vi "Read Spreadsheet Settings all.vi"(11 "Select Data Source":enum16{"auto.csv", "Robot Main"}(ring)) -> (3 "Autonomous Data":T1(array[cluster]))   [LabVIEW 2017]
uses:
  Framework/Robot Global Data.vi
  <vilib>/Utility/file.llb/Read Delimited Spreadsheet (string).vi
panel:
  out "error out":errorcluster
  out "all rows":string[][](array[string])
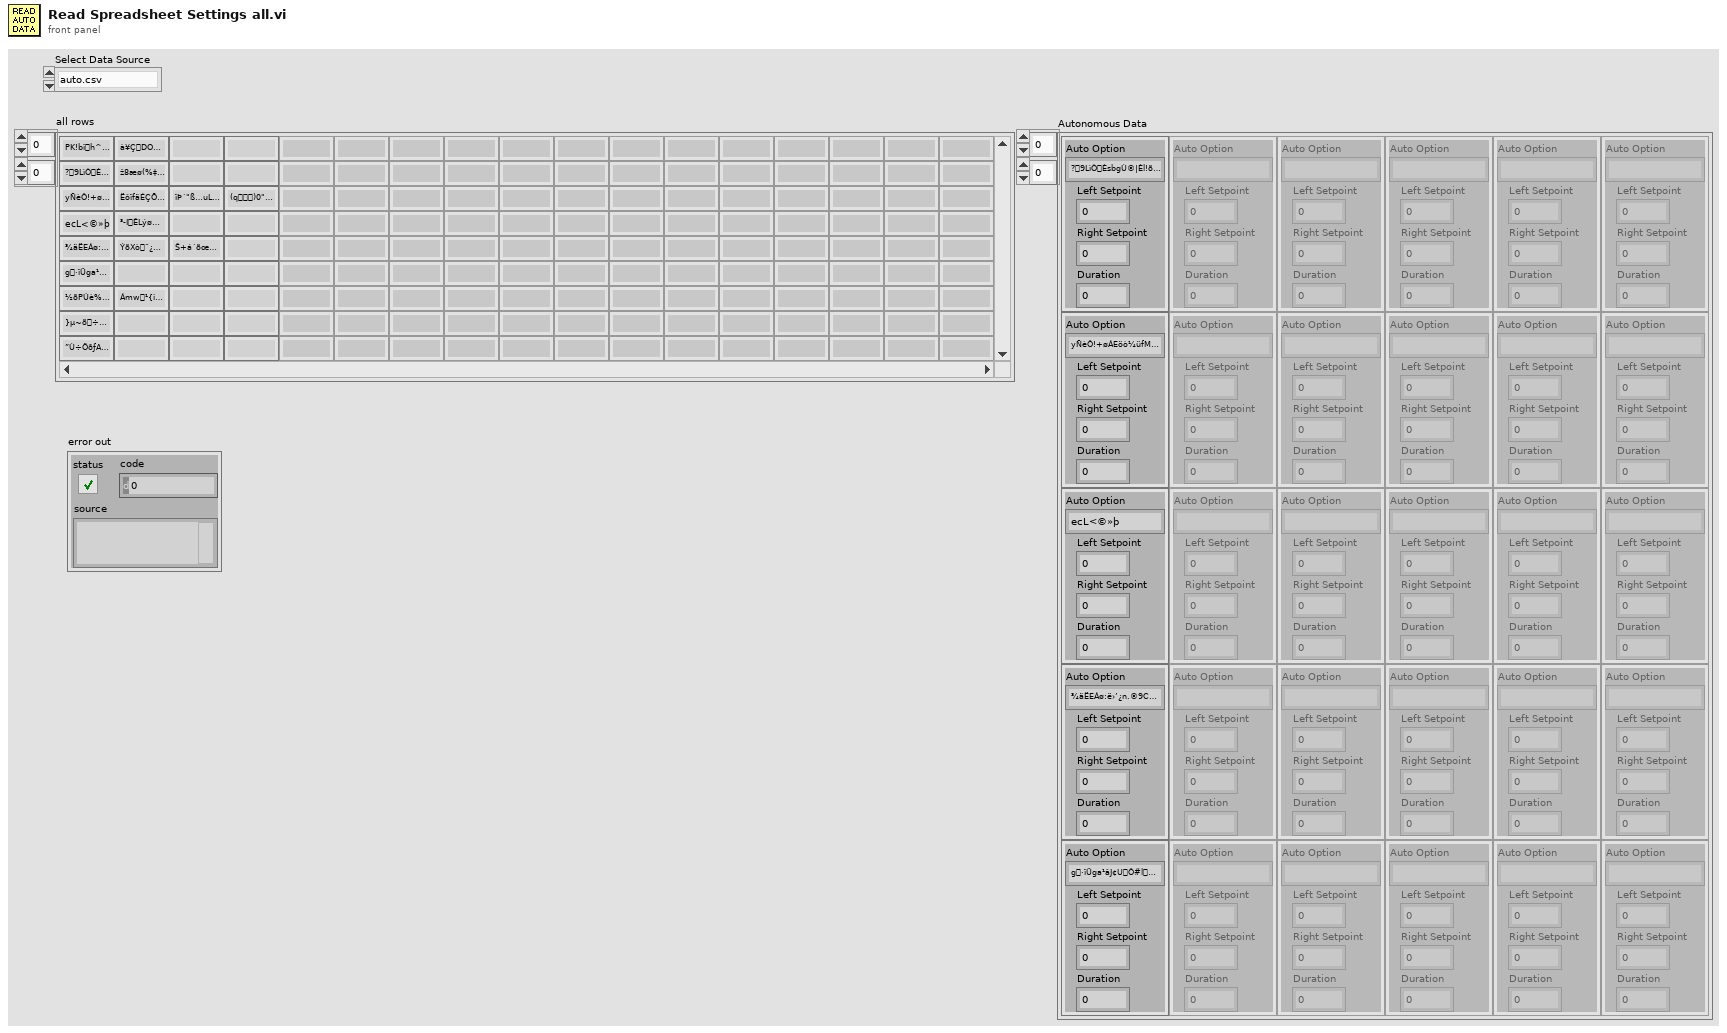
[diagram p1: front panel]
types:
  T1 = cluster{"Auto Option":string, "Left Setpoint":dbl, "Right Setpoint":dbl, "Duration":dbl}[][]
  T2 = cluster{"Auto Option":string, "Left Setpoint":dbl, "Right Setpoint":dbl, "Duration":dbl}
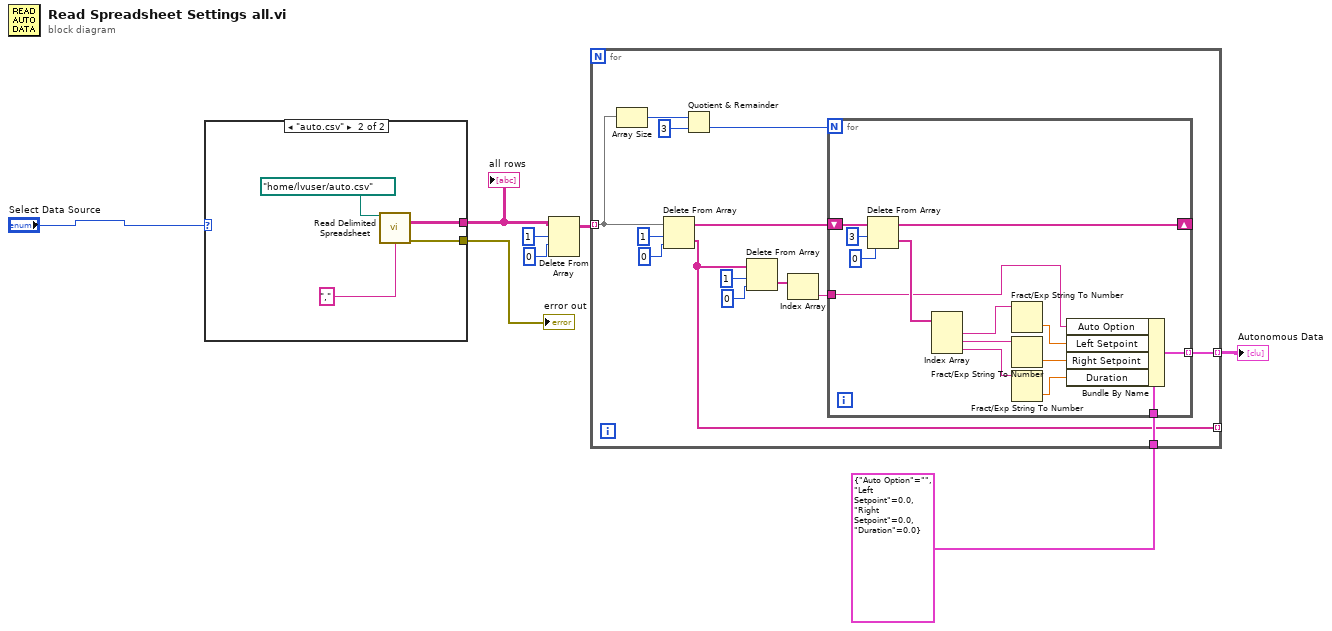
[diagram p0: block diagram]
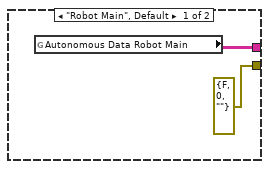
[diagram p2: hidden frame]
diagram:
  n1 = case shown="\"auto.csv\"" "Select Data Source" {
    tunnel: [errorcluster {"status"=FALSE, "code"=0, "source"=""} ("error out") w14] -> w8
    tunnel: [w10 w12] -> w4
    frame "Robot Main", Default {
      n2 = global read "Robot Global Data.vi" "Autonomous Data Robot Main"() -> (w10:string[][])
    }
    frame "auto.csv" {
      n3 = call-poly <vilib>:"Read Delimited Spreadsheet.vi"("file path (dialog if empty)"=path "/home/lvuser/auto.csv" ("Filepath"), "delimiter (\\t)"="," ("delimiter (\\t)")) -> ("all rows"=w12:string[][], "error out"=w14:errorcluster)  [unwired: 8 in, 4 out]
    }
  }
  "all rows" <- w4
  "error out" <- w8
  n4 = Delete From Array(array=w4, length=1, index (row)=0 ("index")) -> (array with subset deleted=w3:string[][])  [unwired: 1 in, 1 out]
  n5 = for {
    tunnel: w3 -> [w23] mode=indexing
    tunnel: T2 {"Auto Option"="", "Left Setpoint"=0.0, "Right Setpoint"=0.0, "Duration"=0.0} -> [w21]
    tunnel: [w20] -> w2 mode=indexing
    tunnel: [w18] -> _ mode=indexing
    n6 = Array Size(array=w23) -> (size(s)=w28:i32)
    n7 = Delete From Array(array=w23, length=1, index=0) -> (deleted portion=w18:string[], array with subset deleted=w22:string[])
    n8 = Quotient & Remainder(x=w28, y=3) -> (floor(x/y)=w26:i32)  [unwired: 1 out]
    n9 = Delete From Array(array=w18, length=1, index=0) -> (deleted portion=w15:string[])  [unwired: 1 out]
    n10 = Index Array(array=w15) -> (element=w16:string)  [unwired: 1 in]
    n11 = for {
      N: w26 -> [_]
      shift-right: [w41] -> _
      shift-left: w22 -> [w42]
      tunnel: w21 -> [w38]
      tunnel: [w30] -> w20 mode=indexing
      tunnel: w16 -> [w29]
      n12 = Delete From Array(array=w42, length=3, index=0) -> (deleted portion=w37:string[], array with subset deleted=w41:string[])
      n13 = Index Array(array=w37) -> (element #1=w36:string, element #2=w35:string, element #3=w34:string)  [unwired: 3 in]
      n14 = Fract/Exp String To Number(string=w36) -> (number=w33:dbl)  [unwired: 3 in, 1 out]
      n15 = Fract/Exp String To Number(string=w35) -> (number=w32:dbl)  [unwired: 3 in, 1 out]
      n16 = Fract/Exp String To Number(string=w34) -> (number=w31:dbl)  [unwired: 3 in, 1 out]
      n17 = Bundle By Name(cluster=w38, "Auto Option"=w29, "Left Setpoint"=w33, "Right Setpoint"=w32, "Duration"=w31) -> (w30:T2)
    }
  }
  "Autonomous Data" <- w2
